vi "WPI_CameraGet Numeric Appearance Property.vi"(8 "error in (no error)":errorcluster, 10 "Property Name":string, 11 "CameraDevRef":T1) -> (0 "error out":errorcluster, 2 "Value":i32, 3 "CameraDevRef dup":T1)   [LabVIEW 2017]
doc: "This software is licensed. Open the labview\\readme\\WPI Robotics Library Open Source License.txt file for more information."
uses:
  <vilib>/Rock Robotics/WPI/Camera/WPI_CameraDevRef.ctl
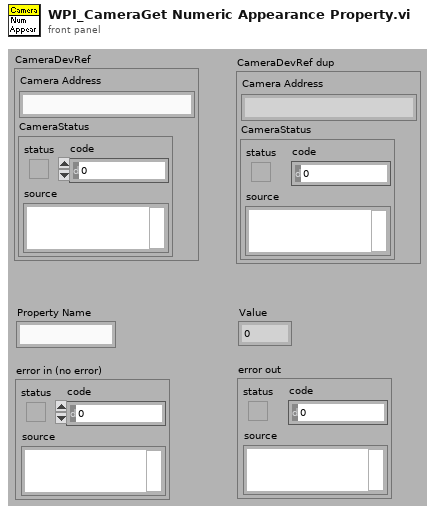
[diagram p1: front panel]
types:
  T1 = typedef "WPI_CameraDevRef.ctl" = cluster{"Camera Address":string, "CameraStatus":errorcluster}
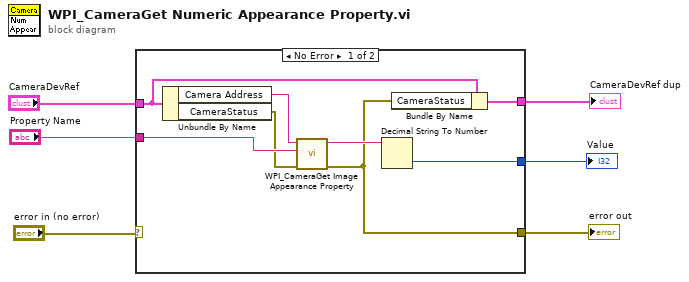
[diagram p0: block diagram]
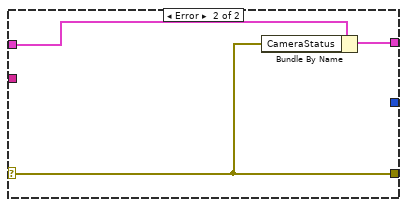
[diagram p2: hidden frame]
diagram:
  n1 = case shown="No Error" "error in (no error)" {
    selector: "error in (no error)" -> [_ w15]
    tunnel: "Property Name" -> [w13 _]
    tunnel: [w11 _] -> w5
    tunnel: [w10 w15] -> w4
    tunnel: "CameraDevRef" -> [w9 w16]
    tunnel: [w8 w17] -> w2
    frame No Error {
      n2 = Unbundle By Name(w9) -> ("Camera Address"=w14:string, "CameraStatus"=w7:errorcluster)
      n3 = call <vilib>:"WPI_CameraGet Image Appearance Property.vi"("error in (no error)"=w7, "Prop String"=w13, "address"=w14) -> ("error out"=w10:errorcluster, "Value"=w12:string)  [unwired: 1 in, 6 out]
      n4 = Decimal String To Number(string=w12) -> (number=w11:i32)  [unwired: 3 out]
      n5 = Bundle By Name(cluster=w9, "CameraStatus"=w10) -> (w8:T1)
    }
    frame Error {
      n6 = Bundle By Name(cluster=w16, "CameraStatus"=w15) -> (w17:T1)
    }
  }
  "error out" <- w4
  "Value" <- w5
  "CameraDevRef dup" <- w2
